vi "Create llb.vi"(7 "Clean Build":bool) -> ()   [LabVIEW 2020]
panel:
  in  "Directories":path[](array[path])=[path "Events for UI Actors/Add RefNum to Actor Data", path "Events for UI Actors/Events for UI Actor Indicators", path "Shortcut Menu Plug-In/Locate in Project", path "Shortcut Menu Plug-In/Open Message Handler", path "Shortcut Menu Plug-In/Move Labels", path "Shortcut Menu Plug-In/Control Visible Toggle", path "Shortcut Menu Plug-In/Add Actor Message", path "Shortcut Menu Plug-In/Convert Node"]
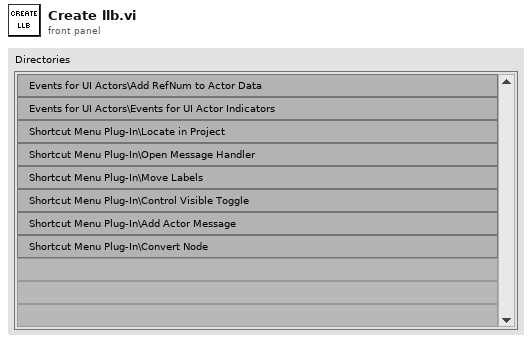
[diagram p1: front panel]
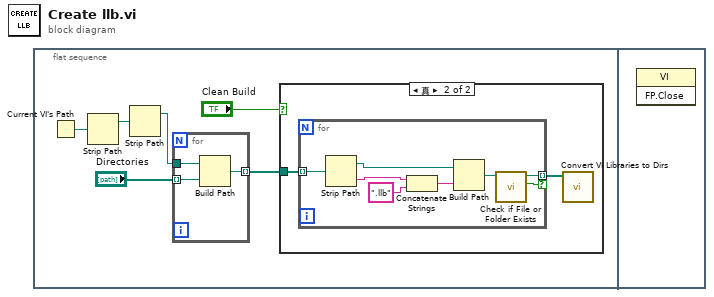
[diagram p0: block diagram]
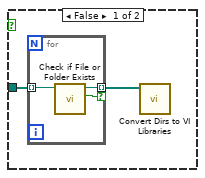
[diagram p2: hidden frame]
diagram:
  n1 = flat-sequence {
    frame #0 {
      n2 = Current VI's Path() -> (path=w6:path)
      n3 = Strip Path(path=w6) -> (stripped path=w5:path)  [unwired: 1 out]
      n4 = Strip Path(path=w5) -> (stripped path=w4:path)  [unwired: 1 out]
      n5 = for {
        tunnel: w4 -> [w24]
        tunnel: "Directories" -> [w23] mode=indexing
        tunnel: [w22] -> w2 mode=indexing
        n6 = Build Path(base path=w24, name or relative path=w23) -> (appended path=w22:path)
      }
      n7 = case shown="真" "Clean Build" {
        tunnel: w2 -> [w8 w13]
        frame False {
          n8 = for {
            tunnel: w8 -> [w11] mode=indexing
            tunnel: [w10] -> w7 mode=indexing if=w9
            n9 = call <vilib>:"Check if File or Folder Exists.vi"("path"=w11) -> ("file or folder exists?"=w9:bool, "dup path"=w10:path)  [unwired: 8 in, 1 out]
          }
          n10 = call "Convert Dirs to VI Libraries.vi"("Directories"=w7) -> ()  [unwired: 11 in]
        }
        frame True {
          n11 = for {
            tunnel: w13 -> [w21] mode=indexing
            tunnel: [w15] -> w12 mode=indexing if=w14
            n12 = Strip Path(path=w21) -> (stripped path=w20:path, name=w19:string)
            n13 = Concatenate Strings(w19, ".llb" ("字符串")) -> (w17:string)
            n14 = Build Path(base path=w20, name or relative path=w17) -> (appended path=w16:path)
            n15 = call <vilib>:"Check if File or Folder Exists.vi"("path"=w16) -> ("file or folder exists?"=w14:bool, "dup path"=w15:path)  [unwired: 8 in, 1 out]
          }
          n16 = call "Convert VI Libraries to Dirs.vi"("VI libraries"=w12) -> ()  [unwired: 8 in, 3 out]
        }
      }
    }
    frame #1 {
      n17 = invoke class="VI" method="FP.Close"() -> ()  [unwired: 3 in, 3 out]
    }
  }
